vi "Waveplate control panel.vi"(4 "PC WP angle":dbl, 5 "Left or right?":dbl(ring)=80.7, 6 "Pump WP angle":dbl, 7 "Waveplate or Pockels cell?":dbl(ring)=55.98 items=["Waveplate"=31.4, "Pockels cell"=76.4], 8 "L/R WP angle":dbl, 9 "Manual?":bool, 10 "Move waveplates":bool, 11 "Home Button":bool) -> (2 "VISA handle out":refnum<visa-resource-name>, 3 "Final positions":dbl[](array[numeric]))   [LabVIEW 2013]
doc: "Demonstrates the fundamentals of the State Machine design pattern in LabVIEW. A state machine, in its simplest form, is a case structure within a while loop, with a state enum wired to a shift register on the loop to define the execution of different cases (or \"states\") of the case structure on different iterations of the loop."
uses:
  Source/State Machine Fundamentals - State Enum.ctl
panel:
  in  "Axis 3\n(Pump)":bool=TRUE
  in  "Axis 2\n(WP/PC)":bool=TRUE
  in  "Axis 1\n(L/R)":bool=TRUE
  in  "Serial port":u8=3
  out "Moving":bool
  out "Initializing":bool
  out "Error out":errorcluster
  out "Moving axis":i32
  in  "Error in":errorcluster
  in  "Stop":bool
  # "Instructions: Start VI. All three SMC100 motion controllers will automatically initialize; this will\ntake several seconds for each and requires homing the stages. Choose waveplate/Pockels cell\nand left/right, OR turn on Manual and set desired angles for each stage. The pump waveplate\nalways uses its manual value. Press Move Waveplates to initiate motion. If any stage gives a \n\"Controller is not in the ready state\" error, it may be necessary to re-initialize by pressing Initialize."
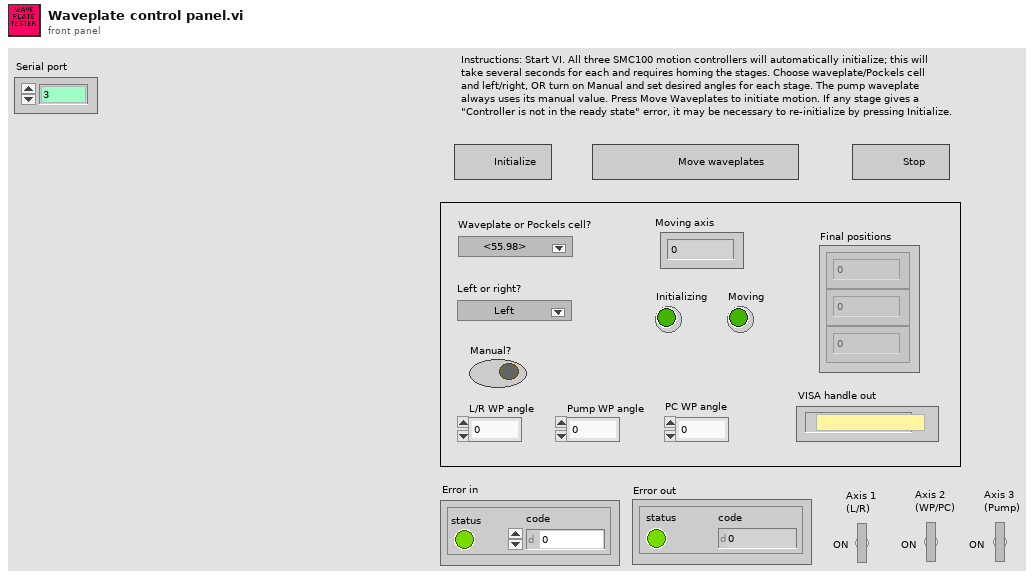
[diagram p1: front panel]
types:
  T1 = typedef "State Machine Fundamentals - State Enum.ctl" = enum16{"Initialize", "Wait for go", "Move", "Stop"}
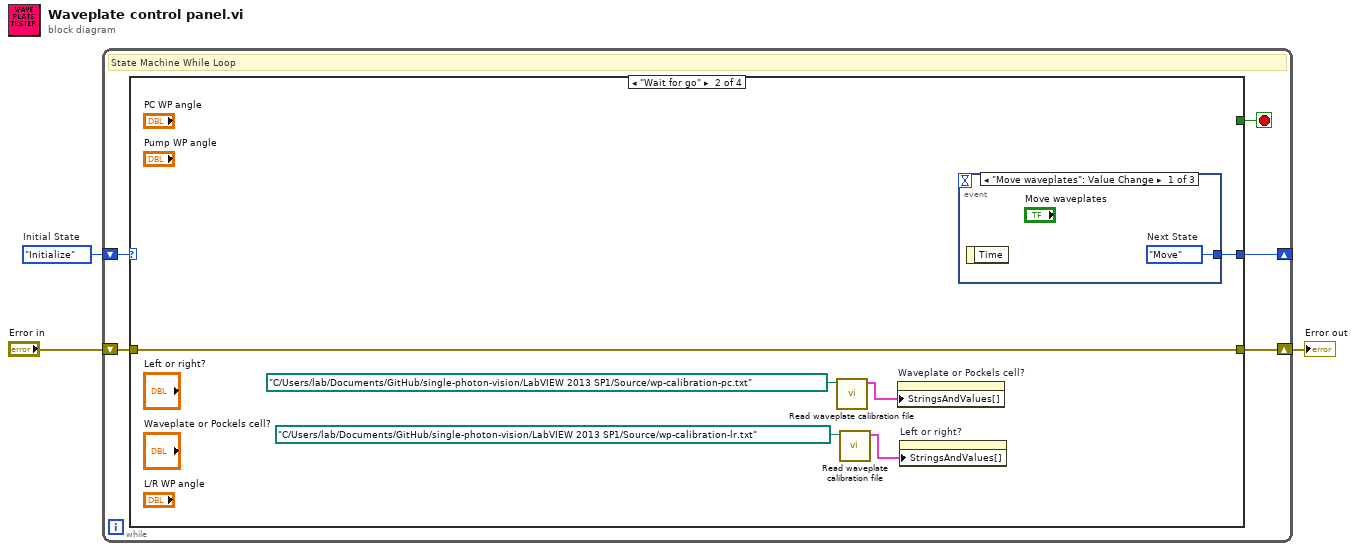
[diagram p0: block diagram]
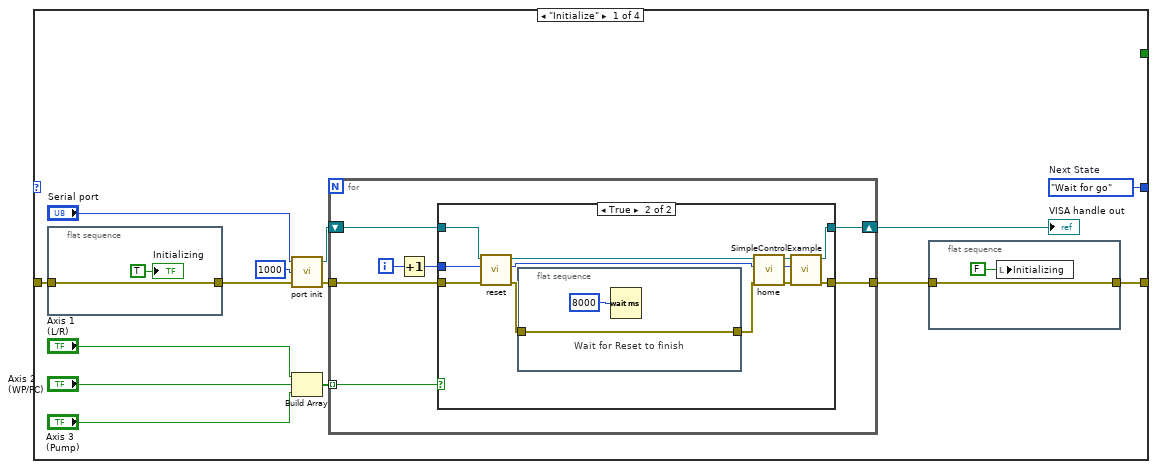
[diagram p2: hidden frame]
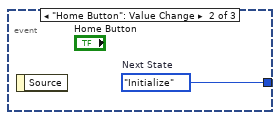
[diagram p4: hidden frame]
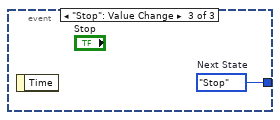
[diagram p5: hidden frame]
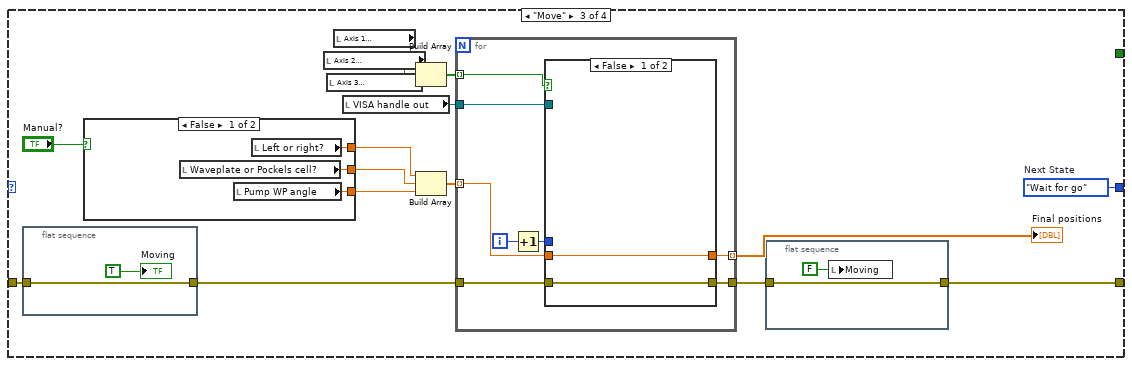
[diagram p6: hidden frame]
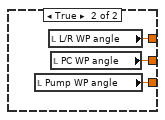
[diagram p7: hidden frame]
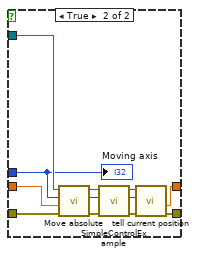
[diagram p8: hidden frame]
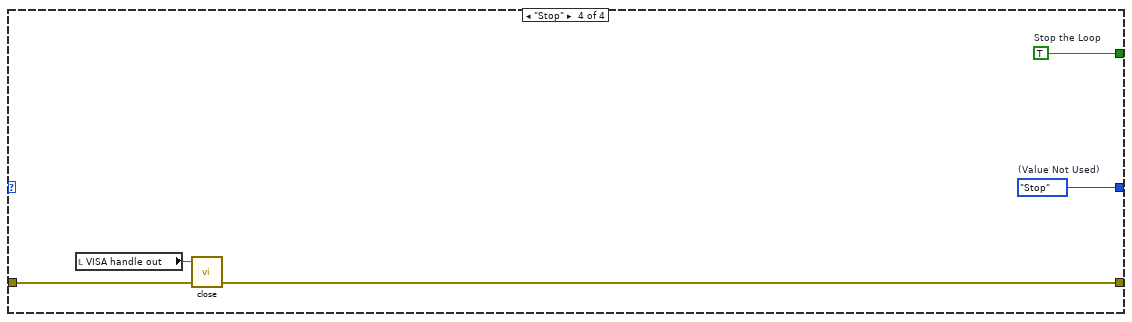
[diagram p9: hidden frame]
diagram:
  w3 = State_Machine_Fundamentals_-_State_Enum."Initialize"  # Initial State
  n1 = while {
    shift-right: [w7] -> _
    shift-left: w3 -> [w8]
    shift-right: [w4] -> w1
    shift-left: "Error in" -> [w5]
    stop <- w6 stop-if-true
    # "State Machine While Loop"
    n2 = case "State Machine Case Structure" shown="\"Wait for go\"" w8 {
      tunnel: [w22 w55 w73 w111] -> w7
      tunnel: [_ _ _ w110] -> w6
      tunnel: w5 -> [w21 w54 w68 w109]
      tunnel: [w20 w54 w65 w108] -> w4
      frame "Initialize" {
        w22 = State_Machine_Fundamentals_-_State_Enum."Wait for go"  # Next State
        n3 = flat-sequence {
          tunnel: w21 -> [w49]
          tunnel: [w49] -> w15
          frame #0 {
            "Initializing" <- TRUE ("Initializing")
          }
        }
        n4 = call "port init.vi"("error in"=w15, "Timeout (ms)"=u32 1000 ("Timeout (300 ms)"), "SerialPort"="Serial port") -> ("error out"=w14:errorcluster, "Visa Handle"=w16:refnum<visa-resource-name>)  [unwired: 1 in]
        n5 = Build Array("Axis 1\n(L/R)", "Axis 2\n(WP/PC)", "Axis 3\n(Pump)") -> (w9:bool[])
        n6 = for {
          tunnel: w14 -> [w27]
          shift-right: [w29] -> w19
          shift-left: w16 -> [w28]
          tunnel: [w26] -> w13
          tunnel: w9 -> [w23] mode=indexing
          i -> [w25]
          n7 = Increment(x=w25) -> (x+1=w24:i32)
          n8 = case shown="True" w23 {
            tunnel: [w31 w36] -> w29
            tunnel: w28 -> [w31 w35]
            tunnel: w27 -> [w30 w34]
            tunnel: [w30 w33] -> w26
            tunnel: w24 -> [_ w32]
            frame False {
            }
            frame True {
              n9 = call "reset.vi"("error in"=w34, "Axis in"=w32, "VISA Handle in"=w35) -> ("error out"=w39:errorcluster, "Axis out"=w40:i32, "VISA Handle out"=w37:refnum<visa-resource-name>)  [unwired: 3 in, 1 out]
              n10 = flat-sequence {
                tunnel: [w44] -> w38
                tunnel: w39 -> [w44]
                frame #0 {
                  # "Wait for Reset to finish"
                  n11 = Wait (ms)(milliseconds to wait=u32 8000) -> ()  [unwired: 1 out]
                }
              }
              n12 = call "home.vi"("error in"=w38, "Axis in"=w40, "VISA Handle in"=w37) -> ("error out"=w42:errorcluster, "Axis out"=w41:i32, "VISA Handle out"=w43:refnum<visa-resource-name>)  [unwired: 3 in, 1 out]
              n13 = call "SimpleControlExample.vi"("error in"=w42, "Axis in"=w41, "VISA Handle in"=w43) -> ("error out"=w33:errorcluster, "VISA Handle out"=w36:refnum<visa-resource-name>)  [unwired: 2 in, 3 out]
            }
          }
        }
        "VISA handle out" <- w19
        n14 = flat-sequence {
          tunnel: w13 -> [w47]
          tunnel: [w47] -> w20
          frame #0 {
            n15 = local write "Initializing"(FALSE ("Initializing")) -> ()
          }
        }
      }
      frame "Wait for go" {
        # "Wait for Event - An Event Structure is used to monitor the user interface for events. In each frame of the Event Structure, the next state of the state machine is specified based on which button was pressed."
        n16 = call "Read waveplate calibration file.vi"("file path (dialog if empty)"=path "C:/Users/lab/Documents/GitHub/single-photon-vision/LabVIEW 2013 SP1/Source/wp-calibration-pc.txt") -> ("Calibration array"=w52:cluster{"String":string, dbl}[])  [unwired: 9 in, 1 out]
        n17 = call "Read waveplate calibration file.vi"("file path (dialog if empty)"=path "C:/Users/lab/Documents/GitHub/single-photon-vision/LabVIEW 2013 SP1/Source/wp-calibration-lr.txt") -> ("Calibration array"=w50:cluster{"String":string, dbl}[])  [unwired: 9 in, 1 out]
        n18 = property on="Waveplate or Pockels cell?" class="Ring (strict)"("StringsAndValues[]"=w52) -> ()  [unwired: 2 in, 2 out]
        n19 = property on="Left or right?" class="Ring (strict)"("StringsAndValues[]"=w50) -> ()  [unwired: 2 in, 2 out]
        n20 = event shown="[0] \"Move waveplates\": Value Change" {
          selector: _ -> [_ _ _]
          dyn-events: _ -> [_ _ _]
          timeout: _ -> [_ _ _]
          tunnel: [w56 w57 w58] -> w55
          event "Move waveplates": Value Change {
            w56 = State_Machine_Fundamentals_-_State_Enum."Move"  # Next State
            n21 = event-data() -> ()  [unwired: 1 in, 1 out]
          }
          event "Home Button": Value Change {
            w57 = State_Machine_Fundamentals_-_State_Enum."Initialize"  # Next State
            n22 = event-data() -> ()  [unwired: 1 in, 1 out]
          }
          event "Stop": Value Change {
            w58 = State_Machine_Fundamentals_-_State_Enum."Stop"  # Next State
            n23 = event-data() -> ()  [unwired: 1 in, 1 out]
          }
        }
      }
      frame "Move" {
        w73 = State_Machine_Fundamentals_-_State_Enum."Wait for go"  # Next State
        # "State 1 - Display a dialog box with a message specific to State 1, then go back to the Wait for Event state."
        n24 = flat-sequence {
          tunnel: w68 -> [w84]
          tunnel: [w84] -> w67
          frame #0 {
            "Moving" <- TRUE ("Moving")
          }
        }
        n25 = case shown="False" "Manual?" {
          tunnel: [w77 w80] -> w71
          tunnel: [w76 w79] -> w70
          tunnel: [w75 w78] -> w63
          frame False {
            n26 = local read "Waveplate or Pockels cell?"() -> (w76:dbl)
            n27 = local read "Pump WP angle"() -> (w75:dbl)
            n28 = local read "Left or right?"() -> (w77:dbl)
          }
          frame True {
            n29 = local read "Pump WP angle"() -> (w78:dbl)
            n30 = local read "L/R WP angle"() -> (w80:dbl)
            n31 = local read "PC WP angle"() -> (w79:dbl)
          }
        }
        n32 = local read "Axis 2\n(WP/PC)"() -> (w61:bool)
        n33 = local read "Axis 3\n(Pump)"() -> (w60:bool)
        n34 = local read "Axis 1\n(L/R)"() -> (w62:bool)
        n35 = local read "VISA handle out"() -> (w69:refnum<visa-resource-name>)
        n36 = Build Array(w62, w61, w60) -> (w59:bool[])
        n37 = Build Array(w71, w70, w63) -> (w72:dbl[])
        n38 = for {
          tunnel: [w92] -> w74 mode=indexing
          tunnel: w67 -> [w91]
          tunnel: [w90] -> w66
          tunnel: w72 -> [w89] mode=indexing
          tunnel: w69 -> [w88]
          tunnel: w59 -> [w87] mode=indexing
          i -> [w86]
          n39 = Increment(x=w86) -> (x+1=w85:i32)
          n40 = case shown="False" w87 {
            tunnel: [w93 w106] -> w92
            tunnel: w91 -> [w94 w105]
            tunnel: [w94 w104] -> w90
            tunnel: w89 -> [w93 w103]
            tunnel: w88 -> [_ w102]
            tunnel: w85 -> [_ w95]
            frame False {
            }
            frame True {
              n41 = call "Move absolute.vi"("error in"=w105, "New target position (units)"=w103, "Axis in"=w95, "VISA Handle in"=w102) -> ("error out"=w96:errorcluster, "Axis out"=w97:i32, "VISA Handle out"=w98:refnum<visa-resource-name>)  [unwired: 2 in, 1 out]
              n42 = call "SimpleControlExample.vi"("error in"=w96, "Axis in"=w97, "VISA Handle in"=w98) -> ("error out"=w99:errorcluster, "Axis out"=w100:i32, "VISA Handle out"=w101:refnum<visa-resource-name>)  [unwired: 2 in, 2 out]
              n43 = call "tell current position.vi"("error in"=w99, "Axis in"=w100, "VISA Handle in"=w101) -> ("error out"=w104:errorcluster, "Current position (units)"=w106:dbl)  [unwired: 2 in, 3 out]
              "Moving axis" <- w95
            }
          }
        }
        "Final positions" <- w74
        n44 = flat-sequence {
          tunnel: w66 -> [w81]
          tunnel: [w81] -> w65
          frame #0 {
            n45 = local write "Moving"(FALSE ("Moving")) -> ()
          }
        }
      }
      frame "Stop" {
        w110 = TRUE  # Stop the Loop
        w111 = State_Machine_Fundamentals_-_State_Enum."Stop"  # (Value Not Used)
        # "Stop - Stop the VI. This is the only state that specifies a TRUE value for the loop conditional terminal."
        n46 = local read "VISA handle out"() -> (w107:refnum<visa-resource-name>)
        n47 = call "close.vi"("error in"=w109, "VISA Handle in"=w107) -> ("error out"=w108:errorcluster)  [unwired: 3 in]
      }
    }
  }
  "Error out" <- w1
